vi "数据发送处理.vi"(1 "PWM":dbl) -> (0 "out":string)   [LabVIEW 2022 SP3]
panel:
  out "floor(x/y)":dbl
  out "x-y*floor(x/y)":dbl
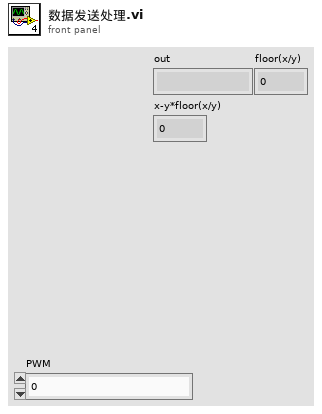
[diagram p1: front panel]
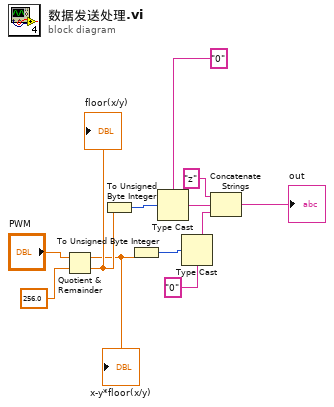
[diagram p0: block diagram]
diagram:
  n1 = Quotient & Remainder(x="PWM", y=256.0) -> (x-y*floor(x/y)=w9:dbl, floor(x/y)=w10:dbl)
  "x-y*floor(x/y)" <- w9
  "floor(x/y)" <- w10
  n2 = To Unsigned Byte Integer(number=w10) -> (unsigned 8bit integer=w7:u8)
  n3 = To Unsigned Byte Integer(number=w9) -> (unsigned 8bit integer=w4:u8)
  n4 = Type Cast(type="0" ("类型"), x=w7) -> (*(type *) &x=w6:string)
  n5 = Type Cast(type="0" ("类型"), x=w4) -> (*(type *) &x=w2:string)
  n6 = Concatenate Strings("z" ("元素"), w6, w2) -> (→"out":string)
